vi "Position Takeoff Button.vi"(8 "error in (no error)":errorcluster, 9 "Slide Refnum":refnum<vi>, 10 "Previous Button Ref":refnum<vi>, 11 "Takeoff Button Ref":refnum<vi>) -> (0 "error out":errorcluster)   [LabVIEW 2014]
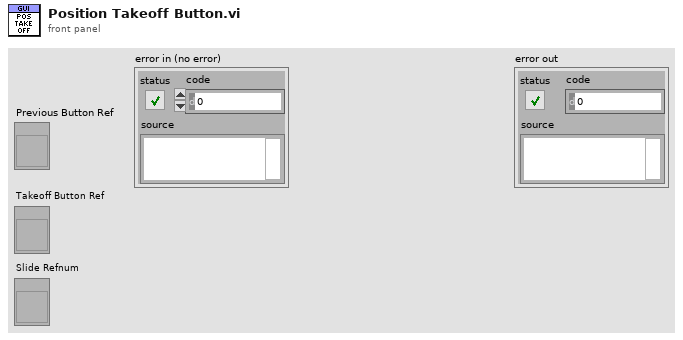
[diagram p1: front panel]
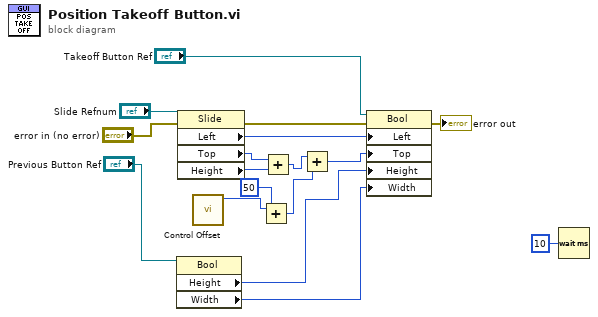
[diagram p0: block diagram]
diagram:
  n1 = property class="Bool"(reference="Previous Button Ref") -> ("Height"=w7:u32, "Width"=w6:u32)  [unwired: 1 in, 2 out]
  n2 = property class="Slide"(reference="Slide Refnum", error in="error in (no error)") -> (error out=w12:errorcluster, "Left"=w10:i32, "Top"=w16:i32, "Height"=w15:u32)  [unwired: 1 out]
  n3 = call "Control Offset.vi"() -> ("Offset From Tab Edge in (px)"=w4:i32)  [unwired: 11 in]
  n4 = Add(x=w4, y=50) -> (x+y=w2:i32)
  n5 = Add(x=w16, y=w15) -> (x+y=w9:u32)
  n6 = Add(x=w9, y=w2) -> (x+y=w8:u32)
  n7 = property class="Bool"(reference="Takeoff Button Ref", error in=w12, "Left"=w10, "Top"=w8, "Height"=w7, "Width"=w6) -> (error out=→"error out":errorcluster)  [unwired: 1 out]
  n8 = Wait (ms)(milliseconds to wait=u32 10) -> ()  [unwired: 1 out]
